vi "cmdElements2Text.vi"(1 "CodeElements":T3={"address"="010000000000", "controlCode"="11", "dataLength"=4.0, "dataSection"="12345678", "checkCode"="7F"}) -> (0 "CommandText":T1)   [LabVIEW 2010]
uses:
  OutputDataFormat.ctl
  <vilib>/xml/Load XML File.vi
  <vilib>/xml/NI_XML.lvlib
  Program Files/National Instruments/LabVIEW 2010/resource/objmgr/DOMUserDefRef.rc
panel:
  out "TextElements":T2
  in  "Path":path=path "D:/MyDocuments/LabviewFiles/CPS/DataIdentityDataBase/ApplicationLayerCommand.xml"
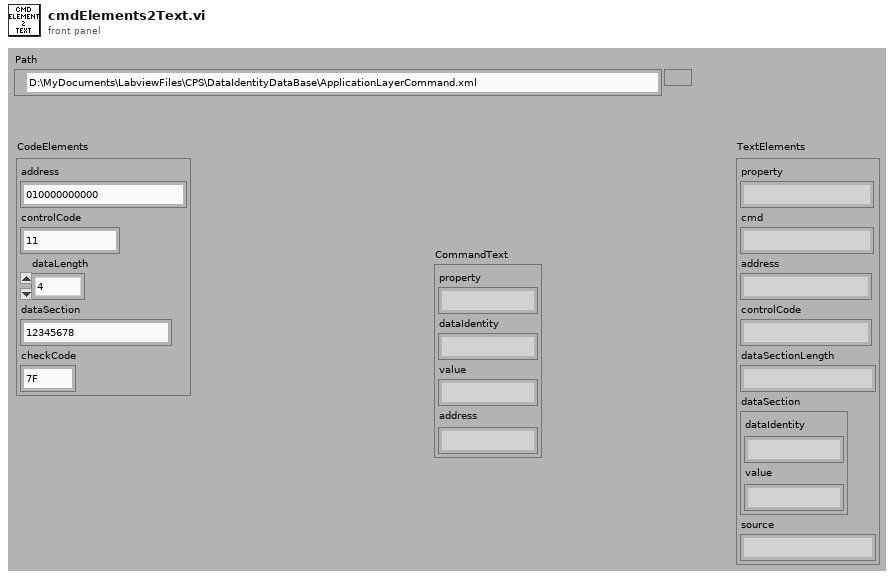
[diagram p1: front panel]
types:
  T1 = typedef "OutputDataFormat.ctl" = cluster{"property":string, "dataIdentity":string, "value":string, "address":string}
  T2 = cluster{"property":string, "cmd":string, "address":string, "controlCode":string, "dataSectionLength":string, "dataSection":cluster{"dataIdentity":string, "value":string}, "source":string}
  T3 = cluster{"address":string, "controlCode":string, "dataLength":dbl, "dataSection":string, "checkCode":string}
  T4 = cluster{"property":string, "cmd":string, "address":string, "controlCode":string, "dataSectionLength":string, "dataSection":string, "source":string}
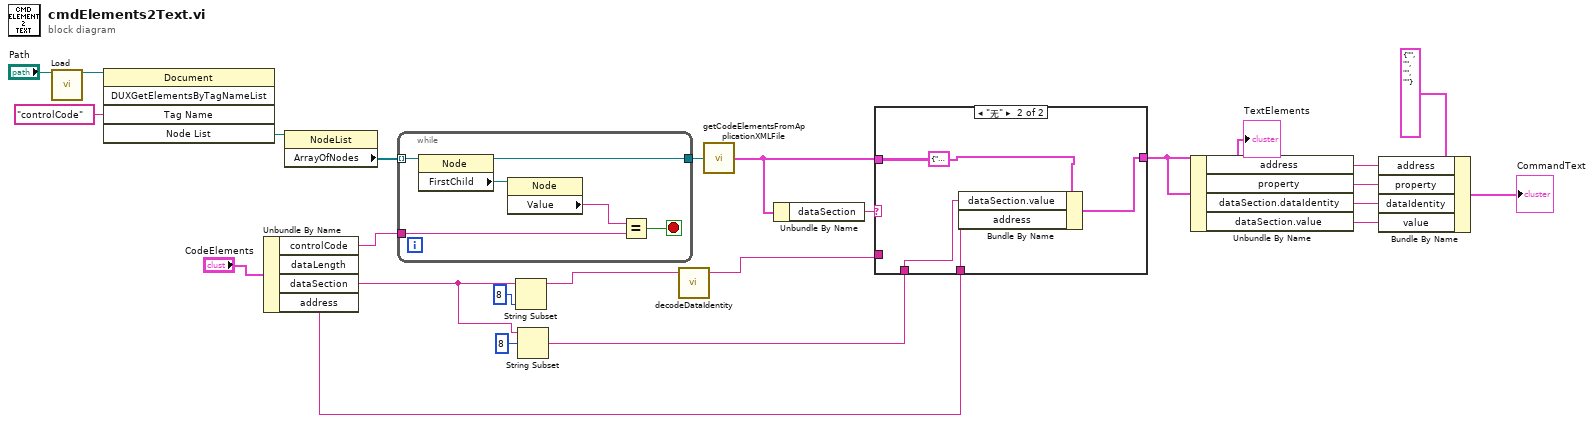
[diagram p0: block diagram]
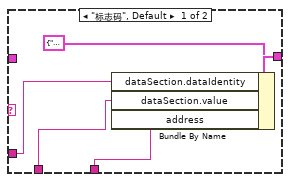
[diagram p2: hidden frame]
diagram:
  n1 = call-poly <vilib>:"Load.vi"("path to XML document"="Path") -> ("DOM document out"=w22:refnum<k20>)  [unwired: 12 in, 2 out]
  n2 = invoke class="Document" method="DUXGetElementsByTagNameList"(reference=w22, "Tag Name"="controlCode") -> ("Node List"=w20:refnum<k20>)  [unwired: 3 in, 4 out]
  n3 = Unbundle By Name("CodeElements") -> ("controlCode"=w19:string, "dataSection"=w8:string, "address"=w14:string)  [unwired: 1 out]
  n4 = property class="NodeList"(reference=w20) -> ("ArrayOfNodes"=w18:refnum<k20>[])  [unwired: 1 in, 2 out]
  n5 = while {
    tunnel: w19 -> [w29]
    tunnel: w18 -> [w30] mode=indexing
    tunnel: [w26] -> w17
    stop <- w27 stop-if-true
    n6 = property class="Node"(reference=w30) -> (reference out=w26:refnum<k20>, "FirstChild"=w25:refnum<k20>)  [unwired: 1 in, 1 out]
    n7 = property class="Node"(reference=w25) -> ("Value"=w28:string)  [unwired: 1 in, 2 out]
    n8 = Equal?(x=w28, y=w29) -> (x = y?=w27:bool)
  }
  n9 = String Subset(string=w8, length (rest)=8 ("offset (0)")) -> (substring=w12:string)  [unwired: 1 in]
  n10 = String Subset(string=w8, offset (0)=8) -> (substring=w7:string)  [unwired: 1 in]
  n11 = call "decodeDataIdentity.vi"("dataIdentityCode"=w12) -> ("dataIdentityText"=w13:string)  [unwired: 4 in]
  n12 = call "getCodeElementsFromApplicationXMLFile.vi"("Node"=w17) -> ("TextElements"=w16:T4)
  n13 = Unbundle By Name(w16) -> ("dataSection"=w15:string)
  n14 = case shown="\"无\"" w15 {
    tunnel: w13 -> [w32 _]
    tunnel: w16 -> [_ _]
    tunnel: [w35 w38] -> w11
    tunnel: w14 -> [w34 w39]
    tunnel: w7 -> [w31 w36]
    frame "标志码", Default {
      n15 = Bundle By Name(cluster=T2 {"property"="读数据", "cmd"="主站请求帧", "address"="AAAAAAAAAAAA", "controlCode"="11", "dataSectionLength"="04", "dataSection"={"dataIdentity"="", "value"=""}, "source"="主站"} ("TextElements"), "dataSection.dataIdentity"=w32, "dataSection.value"=w31, "address"=w34) -> (w35:T2)
    }
    frame "无" {
      n16 = Bundle By Name(cluster=T2 {"property"="读数据", "cmd"="主站请求帧", "address"="AAAAAAAAAAAA", "controlCode"="11", "dataSectionLength"="04", "dataSection"={"dataIdentity"="", "value"=""}, "source"="主站"} ("TextElements"), "dataSection.value"=w36, "address"=w39) -> (w38:T2)
    }
  }
  "TextElements" <- w11
  n17 = Unbundle By Name(w11) -> ("address"=w1:string, "property"=w6:string, "dataSection.dataIdentity"=w5:string, "dataSection.value"=w4:string)
  n18 = Bundle By Name(cluster=T1 {"property"="", "dataIdentity"="", "value"="", "address"=""} ("CommandText"), "address"=w1, "property"=w6, "dataIdentity"=w5, "value"=w4) -> (→"CommandText":T1)
